vi "Add Test Case XML Tag.vi"(8 "error in (no error)":errorcluster, 9 "Test Case Result":cluster{"Name":string, "Case Result":T1}, 10 "Owning Suite":string, 11 "Reports.lvlib:XML Report.lvclass":refnum<class "XML Report.lvclass">) -> (0 "error out":errorcluster, 3 "output cluster":refnum<class "XML Report.lvclass">)   [LabVIEW 2020, in "Reports.lvlib" / "XML Report.lvclass"]
doc: "Add a new element to an existing DOM document."
uses:
  XML Report.lvclass
  Case Result.ctl
  Core/Result/Status.ctl
  XML Report.lvclass/XML Report.ctl
  <resource>/objmgr/DOMUserDefRef.rc
  Core/Result/Result.lvlib
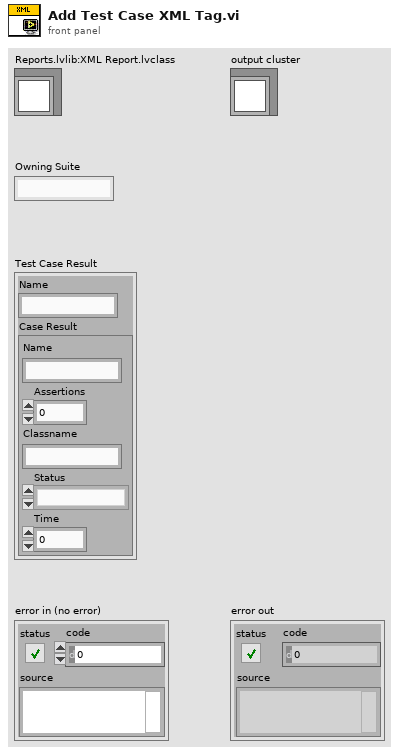
[diagram p1: front panel]
types:
  T1 = typedef "Reports.lvlib/XML Report.lvclass/Case Result.ctl" = cluster{"Name":string, "Assertions":i32, "Classname":string, "Status":T2, "Time":dbl}
  T2 = typedef "Result.lvlib/Status.ctl" = enum16{"", "Passed", "Failed", "Error", "Skipped", "Setup Error", "Broken", "Teardown Error"}
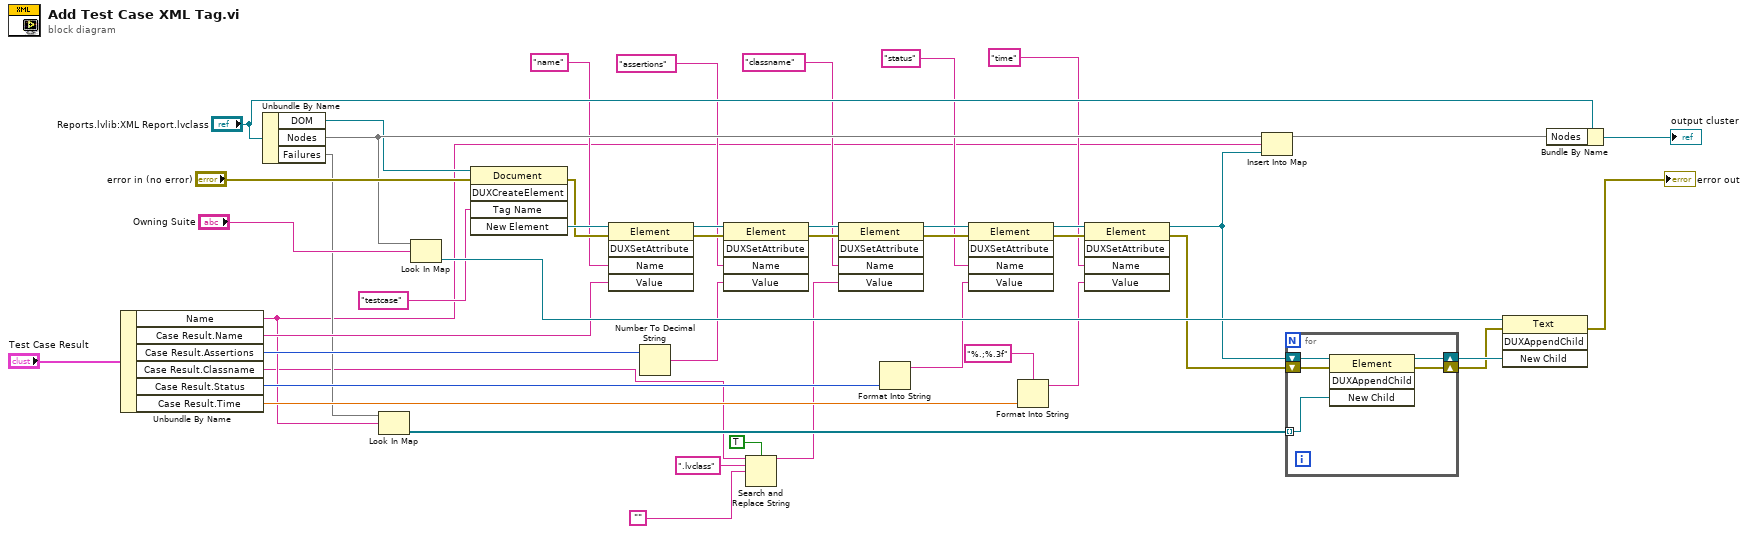
[diagram p0: block diagram]
diagram:
  n1 = Unbundle By Name("Test Case Result") -> ("Name"=w6:string, "Case Result.Name"=w31:string, "Case Result.Assertions"=w28:i32, "Case Result.Classname"=w5:string, "Case Result.Status"=w18:T2, "Case Result.Time"=w14:dbl)
  n2 = Unbundle By Name("Reports.lvlib:XML Report.lvclass") -> ("DOM"=w38:refnum<k20>, "Nodes"=w42:map{string, refnum<k20>}, "Failures"=w7:map{string, refnum<k20>[]})
  n3 = Look In Map(map=w7, key=w6) -> (value=w8:refnum<k20>[])  [unwired: 1 in, 1 out]
  n4 = Look In Map(map=w42, key="Owning Suite") -> (value=w43:refnum<k20>)  [unwired: 1 in, 1 out]
  n5 = invoke class="Document" method="DUXCreateElement"(reference=w38, error in="error in (no error)", "Tag Name"="testcase") -> (error out=w34:errorcluster, "New Element"=w35:refnum<k20>)  [unwired: 2 in, 3 out]
  n6 = invoke class="Element" method="DUXSetAttribute"(reference=w35, error in=w34, "Name"="name", "Value"=w31) -> (reference out=w29:refnum<k20>, error out=w33:errorcluster)  [unwired: 1 in, 3 out]
  n7 = Number To Decimal String(number=w28) -> (decimal integer string=w26:string)  [unwired: 1 in]
  n8 = invoke class="Element" method="DUXSetAttribute"(reference=w29, error in=w33, "Name"="assertions", "Value"=w26) -> (reference out=w24:refnum<k20>, error out=w30:errorcluster)  [unwired: 1 in, 3 out]
  n9 = Search and Replace String(case sensitive?=TRUE ("ignore case? (F)"), input string=w5, search string=".lvclass", replace string="" ("replace string (\"\")")) -> (result string=w4:string)  [unwired: 4 in, 3 out]
  n10 = invoke class="Element" method="DUXSetAttribute"(reference=w24, error in=w30, "Name"="classname", "Value"=w4) -> (reference out=w21:refnum<k20>, error out=w25:errorcluster)  [unwired: 1 in, 3 out]
  n11 = Format Into String(w18) -> (resulting string=w19:string)  [unwired: 3 in, 1 out]
  n12 = invoke class="Element" method="DUXSetAttribute"(reference=w21, error in=w25, "Name"="status", "Value"=w19) -> (reference out=w17:refnum<k20>, error out=w22:errorcluster)  [unwired: 1 in, 3 out]
  n13 = Format Into String(format string="%.;%.3f", w14) -> (resulting string=w13:string)  [unwired: 2 in, 1 out]
  n14 = invoke class="Element" method="DUXSetAttribute"(reference=w17, error in=w22, "Name"="time", "Value"=w13) -> (reference out=w12:refnum<k20>, error out=w9:errorcluster)  [unwired: 1 in, 3 out]
  n15 = Insert Into Map(map in=w42, key=w6, value=w12) -> (map out=w40:map{string, refnum<k20>})  [unwired: 2 out]
  n16 = for {
    shift-right: [w50] -> w11
    shift-left: w12 -> [w51]
    shift-right: [w49] -> w10
    shift-left: w9 -> [w48]
    tunnel: w8 -> [w47] mode=indexing
    n17 = invoke class="Element" method="DUXAppendChild"(reference=w51, error in=w48, "New Child"=w47) -> (reference out=w50:refnum<k20>, error out=w49:errorcluster)  [unwired: 1 in, 2 out]
  }
  n18 = invoke class="Text" method="DUXAppendChild"(reference=w43, error in=w10, "New Child"=w11) -> (error out=→"error out":errorcluster)  [unwired: 1 in, 3 out]
  n19 = Bundle By Name(cluster="Reports.lvlib:XML Report.lvclass", "Nodes"=w40) -> (→"output cluster":refnum<class "XML Report.lvclass">)
